vi "TCP PXI Listener.vi"(11 "error in (no error)":errorcluster) -> (4 "connection ID":refnum<k5>, 8 "Connected?":bool, 15 "error out":errorcluster)   [LabVIEW 2015]
uses:
  DAQ Engine VIs/PXI Globals.vi
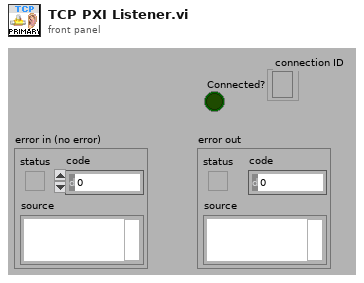
[diagram p1: front panel]
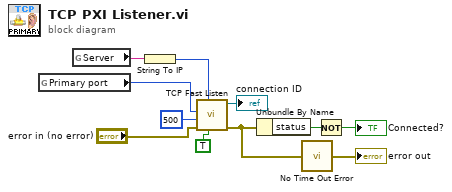
[diagram p0: block diagram]
diagram:
  n1 = global read "PXI Globals.vi" "Primary port"() -> (w7:u16)
  n2 = global read "PXI Globals.vi" "Server"() -> (w5:string)
  n3 = String To IP(1:w5) -> (0:w6:u32)
  n4 = call "TCP Fast Listen.vi"("TCP_NODELAY (true)"=TRUE, "net address"=w6, "error in (no error)"="error in (no error)", "timeout ms (wait forever: -1)"=500, "port"=w7) -> ("error out"=w9:errorcluster, "connection ID"=→"connection ID":refnum<k5>)  [unwired: 3 in, 2 out]
  n5 = Unbundle By Name(w9) -> ("status"=w10:bool)
  n6 = call "No Time Out Error.vi"("error in"=w9) -> ("error out"=→"error out":errorcluster)  [unwired: 14 in]
  n7 = Not(x=w10) -> (.not. x?=→"Connected?":bool)
